vi "mro set Stock Command(incomplete).vi"(8 "error in (no error)":errorcluster, 9 "status":i32, 10 "index":i32, 11 "command":dbl) -> (0 "error out":errorcluster, 1 "status out":i32, 2 "function return":i8, 3 "command out":dbl)   [LabVIEW 2016, in "mirao52e_32bit.lvlib"]
doc: "MIRAOEXPORT MroBoolean MIRAOCALL mro_setStockCommand( \n MroCommand command, \n int index,\n int* status\n );"
uses:
  mirao52e_32bit.lvlib
  mirao52e.dll
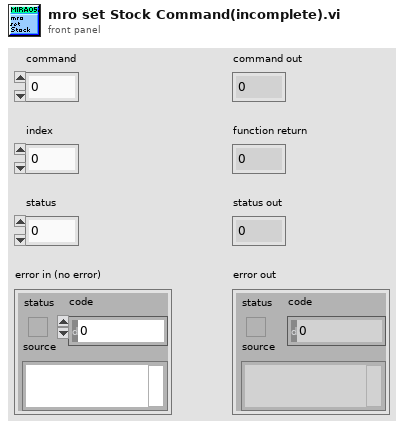
[diagram p1: front panel]
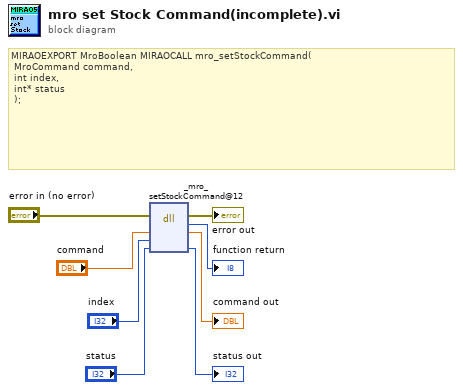
[diagram p0: block diagram]
diagram:
  # "MIRAOEXPORT MroBoolean MIRAOCALL mro_setStockCommand( \n\tMroCommand command, \n\tint index,\n\tint* status\n\t);"
  n1 = dll-call lib="C:/Users/nvladim/Documents/Nikita-MDC/code/LabView/miraoDriver_32bit/mirao52e.*" fn="_mro_setStockCommand@12"(error in="error in (no error)", "command"="command", "index"="index", "status"="status") -> (error out=→"error out":errorcluster, →"function return":i8, "command"=→"command out":dbl, "status"=→"status out":i32)  [unwired: 3 in, 1 out]
